vi "After Launch Init Core.vi"(8 "error in (no error)":errorcluster, 11 "CS++Nanotec in":refnum<class "CS++Nanotec.lvclass">) -> (0 "error out":errorcluster, 3 "CS++Nanotec out":refnum<class "CS++Nanotec.lvclass">)   [LabVIEW 2015, in "CS++Nanotec.lvlib" / "CS++Nanotec.lvclass"]
doc: "Use <b>Pre Launch init.vi</b> method for sanity checks that are supposed to prevent the actor from launching if they fail. Use <B>this</B> method instead to initialize this actor when it has been activated. A corresponding high priority message will become dispatched before the <B>Actor Core.vi</b> is called.\n\n<b>Derived classed should call the parent methode first</b> and their own initialization code after.\n\nRefer also to the ongoing discussion at https://decibel.ni.com/content/message/57394#57394."
uses:
  CS++Nanotec.lvclass
  CSPP_Core/Classes/CS++ProcessVariables/ProcessVariable/PV.lvclass
  CS++Nanotec.lvclass/CS++Nanotec.ctl
  CSPP_Core/Classes/CS++ProcessVariables/ProcessVariable/PV.lvclass/PV.ctl
  CSPP_Core/Classes/CS++ProcessVariables/ProcessVariable/Write Data.vi
  CSPP_Core/Classes/CS++ProcessVariables/ProcessVariable/Write Error.vi
  CSPP_Core/Classes/CS++ProcessVariables/ProcessVariable/Write Quality.vi
  CSPP_Core/Classes/CS++ProcessVariables/ProcessVariable/Write status.vi
  CSPP_Core/Classes/CS++ProcessVariables/ProcessVariable/Write Timestamp.vi
  CSPP_DeviceBase/CS++Motor/CS++Motor.lvclass
  CSPP_Core/Classes/CS++ProcessVariables/PVConnection/PVConnection.lvclass
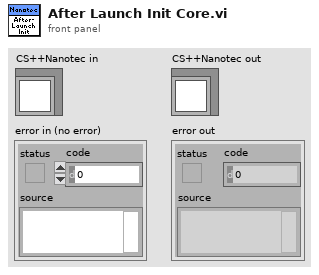
[diagram p1: front panel]
types:
  T1 = cluster{"Read Access":enum8{"Allowed", "Required", "None"}, "Write Access":enum8{"Allowed", "Required", "None"}}
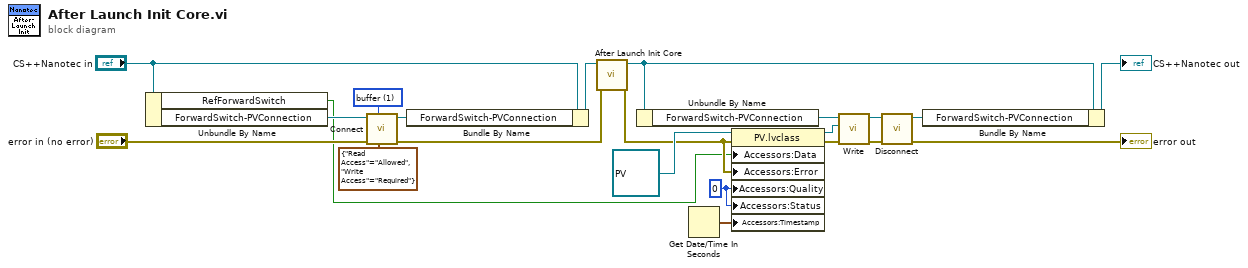
[diagram p0: block diagram]
diagram:
  w6 = 0 ("Quality")
  w16 = u16 1 items=["commit", "buffer"] ("Mode (buffer)")
  n1 = Unbundle By Name("CS++Nanotec in") -> ("RefForwardSwitch"=w1:bool, "ForwardSwitch-PVConnection"=w21:refnum<class "PVConnection.lvclass">)
  n2 = call "Connect.vi"("Access (R/W allowed)"=T1 {"Read Access"=enum."Allowed", "Write Access"=enum."Required"}, "Mode (buffer)"=w16, "Error In"="error in (no error)", "PVConnection in"=w21) -> ("Error Out"=w13:errorcluster, "PVConnection out"=w17:refnum<class "PVConnection.lvclass">)  [unwired: 6 in]
  n3 = Bundle By Name(cluster="CS++Nanotec in", "ForwardSwitch-PVConnection"=w17) -> (w18:refnum<class "CS++Nanotec.lvclass">)
  n4 = call-parent "After Launch Init Core.vi"("error in (no error)"=w13, "CS++Motor in"=w18) -> ("error out"=w2:errorcluster, "CS++Motor out"=w14:refnum<class "CS++Nanotec.lvclass">)  [unwired: 8 in]
  n5 = Unbundle By Name(w14) -> ("ForwardSwitch-PVConnection"=w12:refnum<class "PVConnection.lvclass">)
  n6 = Get Date/Time In Seconds() -> (seconds since 1Jan1904=w7:timestamp)
  n7 = property class="PV.lvclass"(reference=refnum<class "PV.lvclass"> refnum ("CS++ProcessVariables.lvlib:PV.lvclass"), error in=w2, "Accessors:Data"=w1, "Accessors:Error"=w2, "Accessors:Quality"=w6, "Accessors:Status"=w6, "Accessors:Timestamp"=w7) -> (reference out=w3:refnum<class "PV.lvclass">, error out=w4:errorcluster)
  n8 = call "Write.vi"("error in (no error)"=w4, "PV"=w3, "PVConnection in"=w12) -> ("error out"=w19:errorcluster, "PVConnection out"=w11:refnum<class "PVConnection.lvclass">)  [unwired: 7 in]
  n9 = call "Disconnect.vi"("error in (no error)"=w19, "PVConnection in"=w11) -> ("error out"=→"error out":errorcluster, "PVConnection out"=w9:refnum<class "PVConnection.lvclass">)  [unwired: 8 in]
  n10 = Bundle By Name(cluster=w14, "ForwardSwitch-PVConnection"=w9) -> (→"CS++Nanotec out":refnum<class "CS++Nanotec.lvclass">)
